vi "Example.vi"() -> ()   [LabVIEW 2017, in "Examples.lvlib"]
uses:
  <vilib>/Utility/sysdir.llb/System Directory Type.ctl
  Examples.lvlib
panel:
  in  "Path":path
  out "App:Default Data Directory":path
  out "Default Directory":path
  out "Temporary Directory":path
  out "Current VI's Path":path
  out "Application Directory":path
  out "VI Library":path
  out "system directory":path
  in  "system directory type":T1 items=["User Home"=0, "User Desktop"=1, "User Documents"=2, "User Application Data"=3, "User Preferences"=4, "User Temporary"=5, "Public Documents"=6, "Public Application Data"=7, "Public Preferences"=8, "Public Cache"=13, "System Core Libraries"=9, "System Installed Libraries"=10, "Application Files"=11, "Boot Volume Root"=12]
  out "appended path":path
  out "stripped path":path
  out "name":string
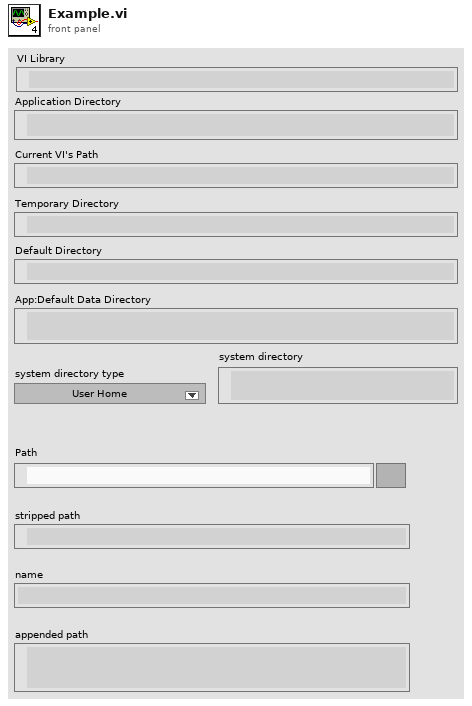
[diagram p1: front panel]
types:
  T1 = typedef "System Directory Type.ctl" = i32
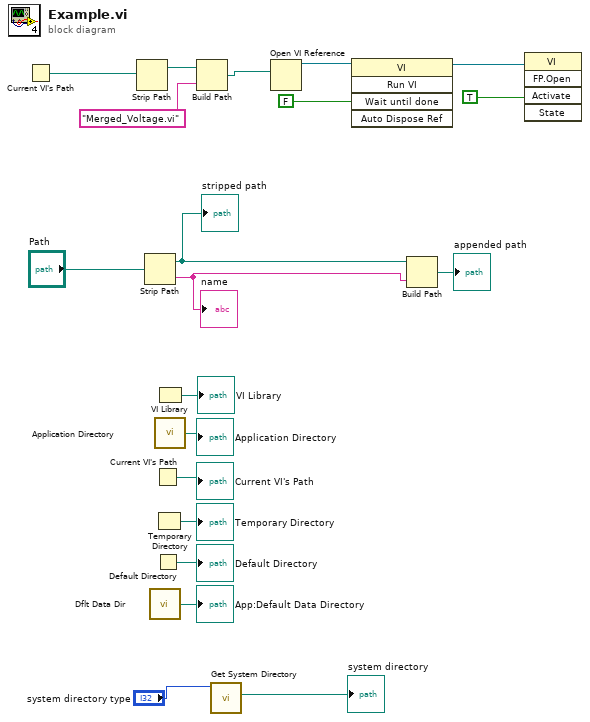
[diagram p0: block diagram]
diagram:
  n1 = Current VI's Path() -> (path=w20:path)
  n2 = Strip Path(path=w20) -> (stripped path=w19:path)  [unwired: 1 out]
  n3 = Strip Path(path="Path") -> (stripped path=w14:path, name=w13:string)
  "name" <- w13
  "stripped path" <- w14
  n4 = call <vilib>:"Dflt Data Dir.vi"() -> ("App:Default Data Directory"=→"App:Default Data Directory":path)
  n5 = Current VI's Path() -> (path=→"Current VI's Path":path)
  n6 = Default Directory() -> (→"Default Directory":path)
  n7 = Temporary Directory() -> (→"Temporary Directory":path)
  n8 = VI Library() -> (path=→"VI Library":path)
  n9 = call <vilib>:"Application Directory.vi"() -> ("Application Directory"=→"Application Directory":path)
  n10 = Build Path(base path=w19, name or relative path="Merged_Voltage.vi") -> (appended path=w3:path)
  n11 = call <vilib>:"Get System Directory.vi"("system directory type"="system directory type") -> ("system directory"=→"system directory":path)  [unwired: 10 in]
  n12 = Open VI Reference(vi path=w3) -> (vi reference=w2:refnum<vi>)  [unwired: 5 in, 1 out]
  n13 = invoke class="VI" method="Run VI"(reference=w2, "Wait until done"=FALSE) -> (reference out=w18:refnum<vi>)  [unwired: 3 in, 4 out]
  n14 = Build Path(base path=w14, name or relative path=w13) -> (appended path=→"appended path":path)
  n15 = invoke class="VI" method="FP.Open"(reference=w18, "Activate"=TRUE) -> ()  [unwired: 3 in, 5 out]
